vi "AprilTagFieldLayout_NewSelect_OLD.vi"(11 "AprilTagField":T1(ring)=enum."2025 Reefscape") -> (3 "AprilTagFieldLayout":T2={"AprilTagMap"={}, "FieldLength"=0.0, "FieldWidth"=0.0, "OriginPosition "=enum."kBlueAllianceWallRightSide,", "OriginPose3d"={"Translation3d"={"X"=0.0, "Y"=0.0, "Z"=0.0}, "Rotation3d"={"Q_quaternion"={"R"=1.0, "V"=[0.0, 0.0, 0.0]}}}} {"OriginPose3d"."Translation3d"."Z" format="%14.3f"; "OriginPose3d"."Translation3d"."Y" format="%14.3f"; "OriginPose3d"."Translation3d"."X" format="%14.3f"})   [LabVIEW 2019, in "Trajectory_Library.lvlib"]
doc: "Define the April Tag field layout based on the input FRC year.\n\nInputs:\n -- AprilTagField -- enum -- Selected Field.\n\nOutputs:\n -- AprilTagFieldLayout -- AprilTagFieldLayout -- Data cluster containing field definition."
uses:
  TypeDef/AprilTagFieldLayout.ctl
  TypeDef/AprilTag.ctl
  TypeDef/POSE3D.ctl
  TypeDef/TRANSLATION3D.ctl
  TypeDef/ROTATION3D.ctl
  TypeDef/QUATERNION.ctl
  Enum/AprilTagFieldLayoutOrignPosition_ENUM.ctl
  AprilTagFieldLayout_New.vi
  Translation3d_Create.vi
  Quaternion_New.vi
  Pose3d_New_Trans3dRot3d.vi
  Rotation3d_Create_Quaternion.vi
  AprilTag_New.vi
  AprilTag_GetAll.vi
  Quaternion_Normalize.vi
  Quaternion_New_Default.vi
  Trajectory_Library.lvlib
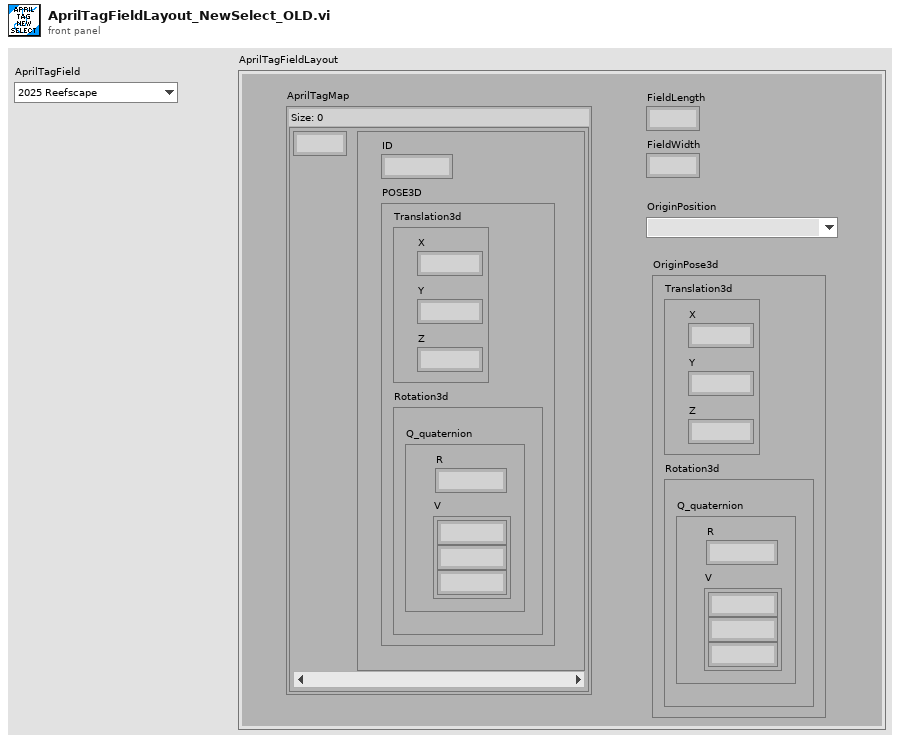
[diagram p1: front panel]
types:
  T1 = enum16{"2022 Rapid React", "2023 Charged Up", "2024 Crescendo", "2025 Reefscape"}
  T2 = typedef "Trajectory_Library.lvlib/AprilTagFieldLayout.ctl" = cluster{"AprilTagMap":map{i32, T3}, "FieldLength":dbl, "FieldWidth":dbl, "OriginPosition ":T8, "OriginPose3d":T4}
  T3 = typedef "Trajectory_Library.lvlib/AprilTag.ctl" = cluster{"ID":i32, "POSE3D":T4}
  T4 = typedef "Trajectory_Library.lvlib/POSE3D.ctl" = cluster{"Translation3d":T5, "Rotation3d":T6}
  T5 = typedef "Trajectory_Library.lvlib/TRANSLATION3D.ctl" = cluster{"X":dbl, "Y":dbl, "Z":dbl}
  T6 = typedef "Trajectory_Library.lvlib/ROTATION3D.ctl" = cluster{"Q_quaternion":T7}
  T7 = typedef "Trajectory_Library.lvlib/QUATERNION.ctl" = cluster{"R":dbl, "V":dbl[]}
  T8 = typedef "Trajectory_Library.lvlib/AprilTagFieldLayoutOrignPosition_ENUM.ctl" = enum16{"kBlueAllianceWallRightSide,", "kRedAllianceWallRightSide,"}
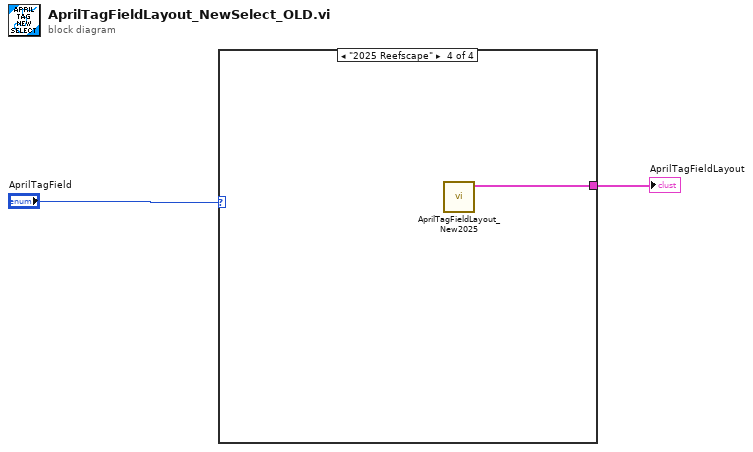
[diagram p0: block diagram]
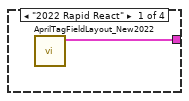
[diagram p2: hidden frame]
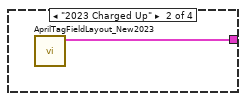
[diagram p3: hidden frame]
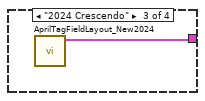
[diagram p4: hidden frame]
diagram:
  n1 = case shown="\"2025 Reefscape\"" "AprilTagField" {
    tunnel: [w3 w4 w5 w6] -> w2
    frame "2022 Rapid React" {
      n2 = call "AprilTagFieldLayout_New2022.vi"() -> ("AprilTagFieldLayout"=w3:T2)  [unwired: 11 in]
    }
    frame "2023 Charged Up" {
      n3 = call "AprilTagFieldLayout_New2023.vi"() -> ("AprilTagFieldLayout"=w4:T2)  [unwired: 11 in]
    }
    frame "2024 Crescendo" {
      n4 = call "AprilTagFieldLayout_New2024.vi"() -> ("AprilTagFieldLayout"=w5:T2)  [unwired: 11 in]
    }
    frame "2025 Reefscape" {
      n5 = call "AprilTagFieldLayout_New2025.vi"() -> ("AprilTagFieldLayout"=w6:T2)  [unwired: 11 in]
    }
  }
  "AprilTagFieldLayout" <- w2
